vi "String_to_num (SubVI).vi"(0 "String in":string, 2 "error in":errorcluster) -> (6 "Rest of string OUT":string, 7 "error out":errorcluster, 9 "output cluster \nof coefficients":T1 {"k1" format="%#_16g"; "k2" format="%#_16g"; "k3" format="%#_16g"; "k4" format="%#_16g"; "k5" format="%#_16g"; "k6" format="%#_16g"; "k7" format="%#_16g"; "R" format="%#_16g"})   [LabVIEW 8.6]
panel:
  out "k4":ext
  out "R":ext
  out "k7":ext
  out "k6":ext
  out "k5":ext
  out "k3":ext
  out "k2":ext
  out "k1":ext
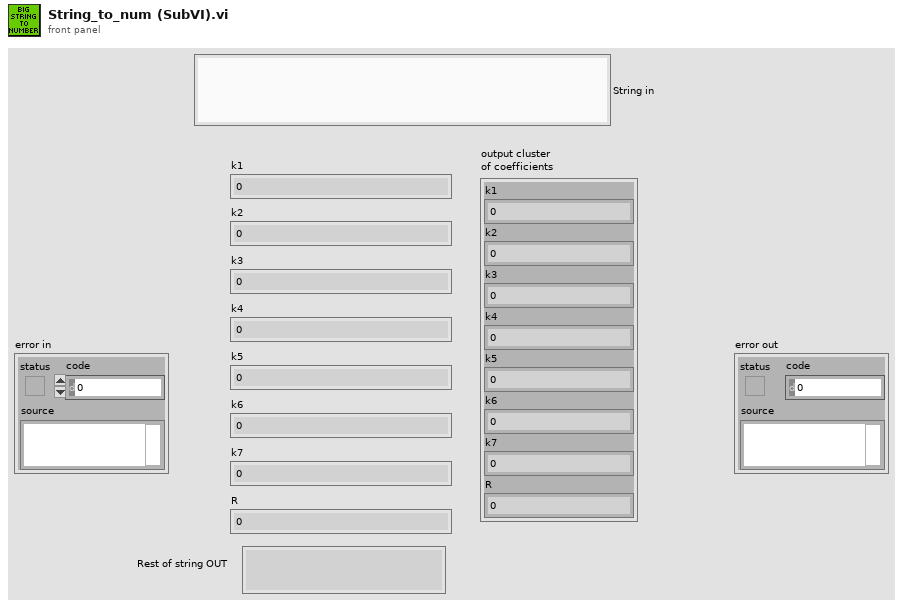
[diagram p1: front panel]
types:
  T1 = cluster{"k1":ext, "k2":ext, "k3":ext, "k4":ext, "k5":ext, "k6":ext, "k7":ext, "R":ext}
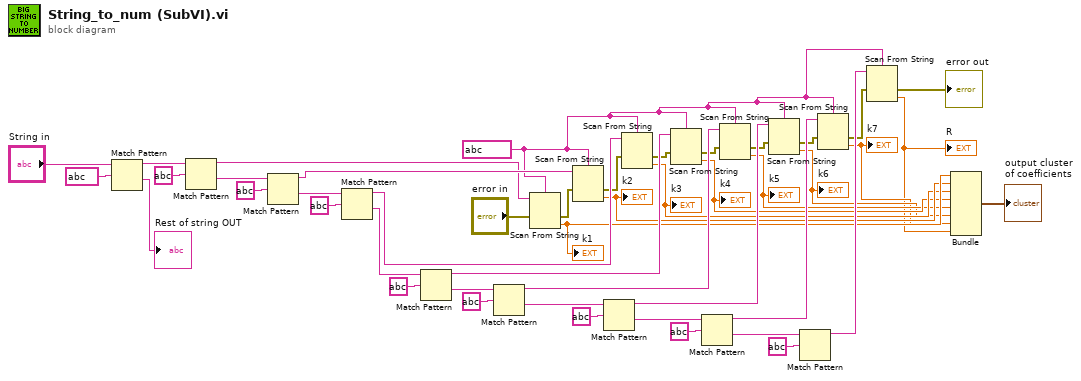
[diagram p0: block diagram]
diagram:
  w13 = string ? ("format string")
  n1 = Match Pattern(string="String in", regular expression=string ?) -> (before substring=w31:string, after substring=→"Rest of string OUT":string)  [unwired: 1 in, 2 out]
  n2 = Match Pattern(string=w31, regular expression=string ? ("delimiter (Tab)")) -> (before substring=w1:string, after substring=w39:string)  [unwired: 1 in, 2 out]
  n3 = Match Pattern(string=w39, regular expression=string ? ("delimiter (Tab)")) -> (before substring=w27:string, after substring=w32:string)  [unwired: 1 in, 2 out]
  n4 = Match Pattern(string=w32, regular expression=string ? ("delimiter (Tab)")) -> (before substring=w26:string, after substring=w33:string)  [unwired: 1 in, 2 out]
  n5 = Match Pattern(string=w33, regular expression=string ? ("delimiter (Tab)")) -> (before substring=w25:string, after substring=w34:string)  [unwired: 1 in, 2 out]
  n6 = Match Pattern(string=w34, regular expression=string ? ("delimiter (Tab)")) -> (before substring=w24:string, after substring=w35:string)  [unwired: 1 in, 2 out]
  n7 = Scan From String(format string=w13, input string=w1, error in="error in") -> (error out=w20:errorcluster, output 1=w10:ext)  [unwired: 2 in, 2 out]
  "k1" <- w10
  n8 = Scan From String(format string=w13, input string=w27, error in=w20) -> (error out=w19:errorcluster, output 1=w9:ext)  [unwired: 2 in, 2 out]
  "k2" <- w9
  n9 = Match Pattern(string=w35, regular expression=string ? ("delimiter (Tab)")) -> (before substring=w23:string, after substring=w36:string)  [unwired: 1 in, 2 out]
  n10 = Scan From String(format string=w13, input string=w26, error in=w19) -> (error out=w18:errorcluster, output 1=w8:ext)  [unwired: 2 in, 2 out]
  "k3" <- w8
  n11 = Scan From String(format string=w13, input string=w25, error in=w18) -> (error out=w17:errorcluster, output 1=w7:ext)  [unwired: 2 in, 2 out]
  "k4" <- w7
  n12 = Match Pattern(string=w36, regular expression=string ? ("delimiter (Tab)")) -> (before substring=w22:string, after substring=w37:string)  [unwired: 1 in, 2 out]
  n13 = Scan From String(format string=w13, input string=w24, error in=w17) -> (error out=w16:errorcluster, output 1=w6:ext)  [unwired: 2 in, 2 out]
  "k5" <- w6
  n14 = Scan From String(format string=w13, input string=w23, error in=w16) -> (error out=w15:errorcluster, output 1=w5:ext)  [unwired: 2 in, 2 out]
  "k6" <- w5
  n15 = Match Pattern(string=w37, regular expression=string ? ("delimiter (Tab)")) -> (before substring=w21:string)  [unwired: 1 in, 3 out]
  n16 = Scan From String(format string=w13, input string=w22, error in=w15) -> (error out=w14:errorcluster, output 1=w4:ext)  [unwired: 2 in, 2 out]
  "k7" <- w4
  n17 = Scan From String(format string=w13, input string=w21, error in=w14) -> (error out=→"error out":errorcluster, output 1=w3:ext)  [unwired: 2 in, 2 out]
  "R" <- w3
  n18 = Bundle("k1"=w10, "k2"=w9, "k3"=w8, "k4"=w7, "k5"=w6, "k6"=w5, "k7"=w4, "R"=w3) -> (→"output cluster \nof coefficients":T1)  [unwired: 1 in]
